vi "unbuffered_xy_graph.vi"() -> ()   [LabVIEW 2019]
panel:
  out "XY Graph":cluster{i32[], i32[]}(graph)
  in  "stop":bool
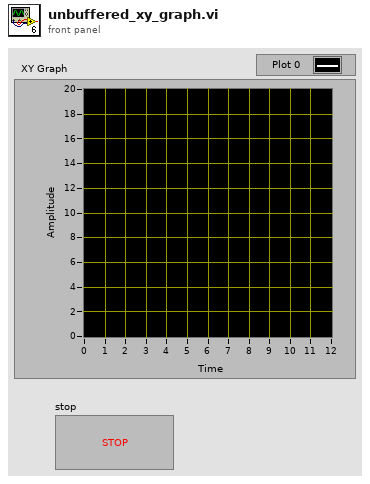
[diagram p1: front panel]
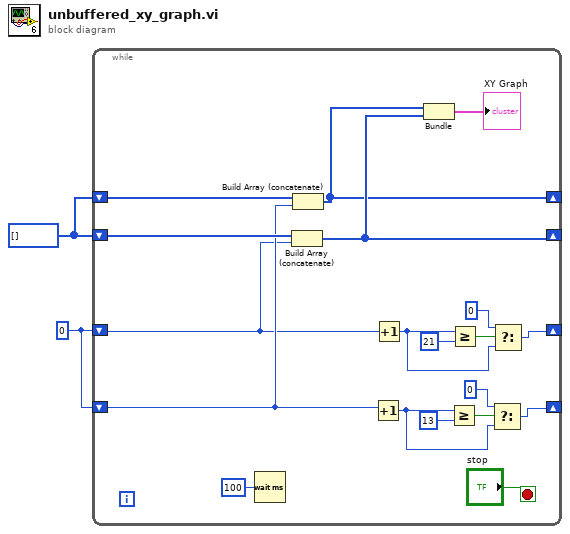
[diagram p0: block diagram]
diagram:
  w2 = i32[] []
  w1 = 0
  n1 = while {
    shift-right: [w17] -> _
    shift-left: w1 -> [w3]
    shift-right: [w11] -> _
    shift-left: w2 -> [w15]
    shift-right: [w4] -> _
    shift-left: w2 -> [w12]
    shift-right: [w6] -> _
    shift-left: w1 -> [w5]
    stop <- "stop" stop-if-true
    n2 = Wait (ms)(milliseconds to wait=u32 100) -> ()  [unwired: 1 out]
    n3 = Build Array (concatenate)(w15, w3) -> (w11:i32[])
    n4 = Build Array (concatenate)(w12, w5) -> (w4:i32[])
    n5 = Increment(x=w5) -> (x+1=w10:i32)
    n6 = Increment(x=w3) -> (x+1=w18:i32)
    n7 = Bundle(w4, w11) -> (→"XY Graph":cluster{i32[], i32[]})  [unwired: 1 in]
    n8 = Greater Or Equal?(x=w10, y=13) -> (x >= y?=w8:bool)
    n9 = Greater Or Equal?(x=w18, y=21) -> (x >= y?=w20:bool)
    n10 = Select(t=0 ("y"), s=w8, f=w10) -> (s? t:f=w6:i32)
    n11 = Select(t=0 ("y"), s=w20, f=w18) -> (s? t:f=w17:i32)
  }
